vi "Console_FPGA_myRIO.vi"() -> ()   [LabVIEW 2017]
uses:
  <vilib>/rvi/Emulation/niFpgaGetClockAttributes.vi
  <vilib>/rvi/Emulation/niFpgaSctlEmulationGetInTimedLoop.vi
  <vilib>/rvi/Emulation/niFpgaEmulationReportErrorSimple.vi
  <vilib>/rvi/Emulation/niFpgaCriticalErrorInLSC.vi
panel:
  out "Position_Z":i16
  out "Position_Y":i16
  out "Position_X":i16
  in  "Reset_Z":bool
  in  "Reset_Y":bool
  in  "Reset_X":bool
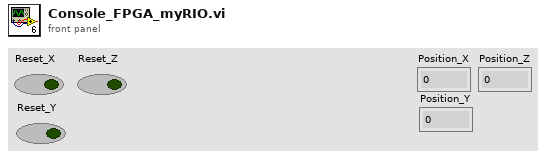
[diagram p1: front panel]
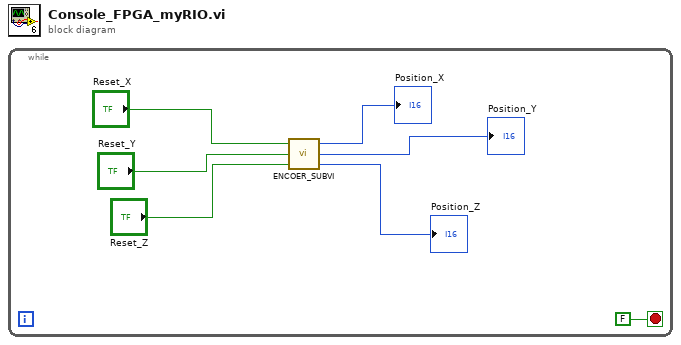
[diagram p0: block diagram]
diagram:
  n1 = while {
    stop <- FALSE stop-if-true
    n2 = call "ENCOER_SUBVI.vi"("Reset_Z"="Reset_Z", "Reset_Y"="Reset_Y", "Reset_X"="Reset_X") -> ("Position_Z"=→"Position_Z":i16, "Position_Y"=→"Position_Y":i16, "Position_X"=→"Position_X":i16)
  }
